vi "Initialize Minimum.vi"(8 "error in (no error)":errorcluster, 11 "Numeric Data Type in":refnum<class "Numeric Data Type.lvclass">) -> (0 "error out":errorcluster, 3 "Numeric Data Type (dup)":refnum<class "Numeric Data Type.lvclass">)   [LabVIEW 2018, in "Numeric Data Type.lvclass"]
uses:
  Numeric Data Type.lvclass
  Numeric Data Type.lvclass/Numeric Data Type.ctl
  Reference Minimum.vi
  Reference Minimum Time.vi
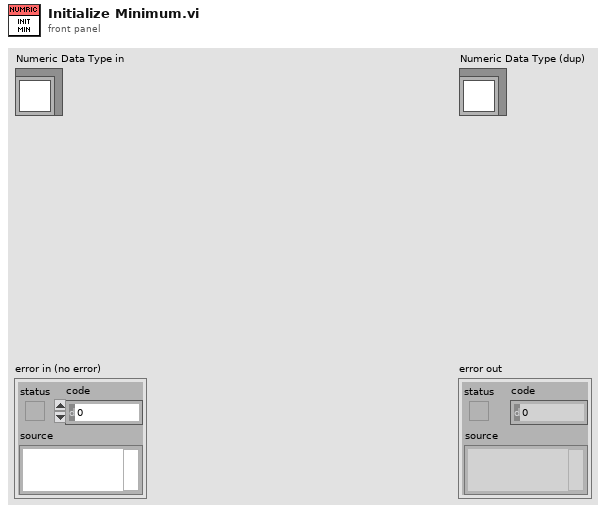
[diagram p1: front panel]
types:
  T1 = typedef "Numeric Data Type.lvclass/Representation Enum.ctl" = enum16{"Extended (EXT)", "Double (DBL)", "Single (SGL)", "Fixed-Point (FXP)", "Quad Integer (I64)", "Long Integer (I32)", "Word Integer (I16)", "Byte Integer (I8)", "Unsigned Quad (U64)", "Unsigned Long (U32)", "Unsigned Word (U16)", "Unsigned Byte (U8)", "Complex Extended (CXT)", "Complex Double (CDB)", "Complex Single (CSG)"}
  T2 = enum8{"Enabled", "Disabled", "Disabled and Grayed Out"}
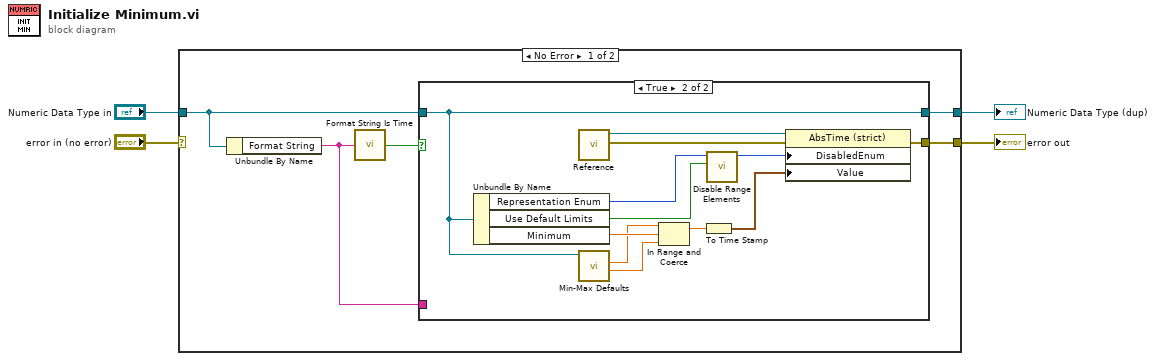
[diagram p0: block diagram]
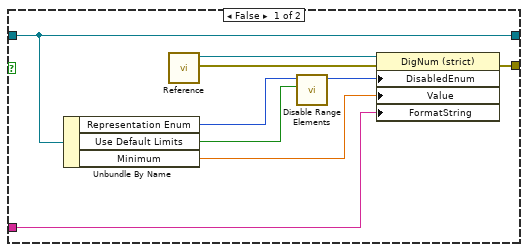
[diagram p2: hidden frame]
diagram:
  n1 = case shown="No Error" "error in (no error)" {
    selector: "error in (no error)" -> [_ w32]
    tunnel: [w9 w32] -> w3
    tunnel: [w8 w31] -> w1
    tunnel: "Numeric Data Type in" -> [w7 w31]
    frame No Error {
      n2 = Unbundle By Name(w7) -> ("Format String"=w5:string)
      n3 = call "Format String Is Time.vi"("Format String"=w5) -> ("Time?"=w6:bool)
      n4 = case shown="True" w6 {
        tunnel: w7 -> [w11 w21]
        tunnel: [w12 w25] -> w9
        tunnel: [w11 w21] -> w8
        tunnel: w5 -> [w10 _]
        frame False {
          n5 = Unbundle By Name(w11) -> ("Representation Enum"=w15:T1, "Use Default Limits"=w14:bool, "Minimum"=w16:dbl)
          n6 = call-poly "Reference.vi"() -> ("error out"=w18:errorcluster, "Minimum"=w17:refnum<vi>)  [unwired: 10 in]
          n7 = call "Disable Range Elements.vi"("Use Default Limits"=w14, "Representation Enum"=w15) -> ("Disabled?"=w13:T2)  [unwired: 9 in]
          n8 = property class="DigNum (strict)"(reference=w17, error in=w18, "DisabledEnum"=w13, "Value"=w16, "FormatString"=w10) -> (error out=w12:errorcluster)  [unwired: 1 out]
        }
        frame True {
          n9 = Unbundle By Name(w21) -> ("Representation Enum"=w28:T1, "Use Default Limits"=w27:bool, "Minimum"=w24:dbl)
          n10 = call-poly "Reference.vi"() -> ("error out"=w30:errorcluster, "Minimum Time"=w29:refnum<vi>)  [unwired: 10 in]
          n11 = call "Min-Max Defaults.vi"("Numeric Data Type in"=w21) -> ("Maximum"=w19:dbl, "Minimum"=w20:dbl)  [unwired: 6 in, 3 out]
          n12 = In Range and Coerce(upper limit=w20, x=w24, lower limit=w19) -> (coerced(x)=w22:dbl)  [unwired: 1 out]
          n13 = To Time Stamp(1:w22) -> (0:w23:timestamp)
          n14 = call "Disable Range Elements.vi"("Use Default Limits"=w27, "Representation Enum"=w28) -> ("Disabled?"=w26:T2)  [unwired: 9 in]
          n15 = property class="AbsTime (strict)"(reference=w29, error in=w30, "DisabledEnum"=w26, "Value"=w23) -> (error out=w25:errorcluster)  [unwired: 1 out]
        }
      }
    }
    frame Error {
    }
  }
  "error out" <- w3
  "Numeric Data Type (dup)" <- w1
